vi "Perform Action.vi"(8 "error in":errorcluster, 11 "Host Measure and Stimulus Subsystems in":refnum<class "Host Measure and Stimulus Subsystems.lvclass">) -> (0 "error out":errorcluster, 3 "Host Measure and Stimulus Subsystems out":refnum<class "Host Measure and Stimulus Subsystems.lvclass">)   [LabVIEW 2023, in "HAL GOOP4.lvlib" / "Host Measure and Stimulus Subsystems.lvclass"]
uses:
  Host Measure and Stimulus Subsystems.lvclass
  Host Measure and Stimulus Subsystems.lvclass/Host Measure and Stimulus Subsystems.ctl
  <vilib>/Utility/error.llb/Error Cluster From Error Code.vi
  <vilib>/ErrorRing/Error Ring.xnode
  Virtual Instrument Base/Virt Instr Base.lvclass
panel:
  out "Output":variant
  in  "Input":variant
  in  "Target Ident":string
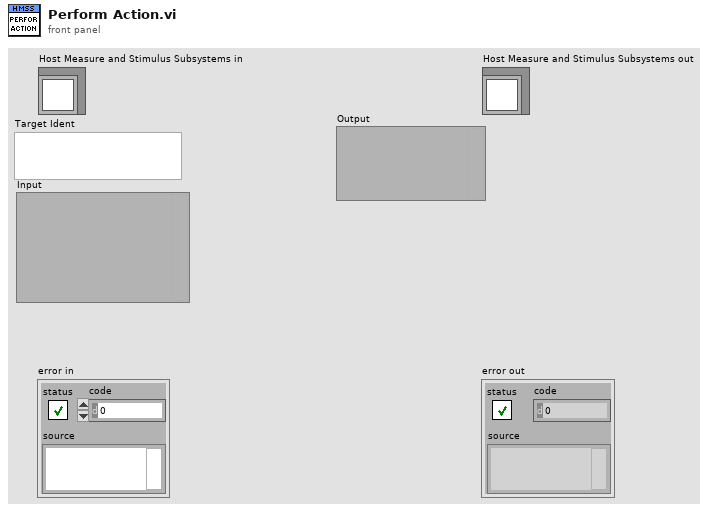
[diagram p1: front panel]
types:
  T1 = map{string, refnum<class "Virt Instr Base.lvclass">}
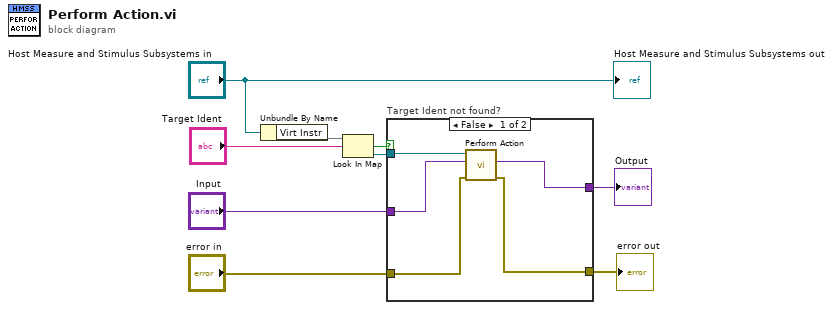
[diagram p0: block diagram]
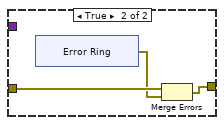
[diagram p2: hidden frame]
diagram:
  n1 = Unbundle By Name("Host Measure and Stimulus Subsystems in") -> ("Virt Instr"=w9:T1)
  n2 = Look In Map(map=w9, key="Target Ident") -> (key not found?=w7:bool, value=w6:refnum<class "Virt Instr Base.lvclass">)  [unwired: 1 in]
  n3 = case "Target Ident not found?" shown="False" w7 {
    tunnel: "error in" -> [w11 w17]
    tunnel: w6 -> [w14 _]
    tunnel: [w10 w15] -> w2
    tunnel: [w13 _] -> w3
    tunnel: "Input" -> [w12 _]
    frame False {
      n4 = call-dynamic "Perform Action.vi"("error in (no error)"=w11, "Input"=w12, "Virt Instrument Base in"=w14) -> ("error out"=w10:errorcluster, "Output"=w13:variant)  [unwired: 6 in, 1 out]
    }
    frame True {
      n5 = xnode "Error Ring"() -> ("error out"=w16:errorcluster)
      n6 = Merge Errors(w17, w16) -> (w15:errorcluster)
    }
  }
  "error out" <- w2
  "Output" <- w3
  "Host Measure and Stimulus Subsystems out" <- "Host Measure and Stimulus Subsystems in"
